vi "이벤트.vi"() -> ()   [LabVIEW 2020]
panel:
  in  "정지":bool
  in  "확인 버튼":bool
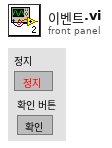
[diagram p1: front panel]
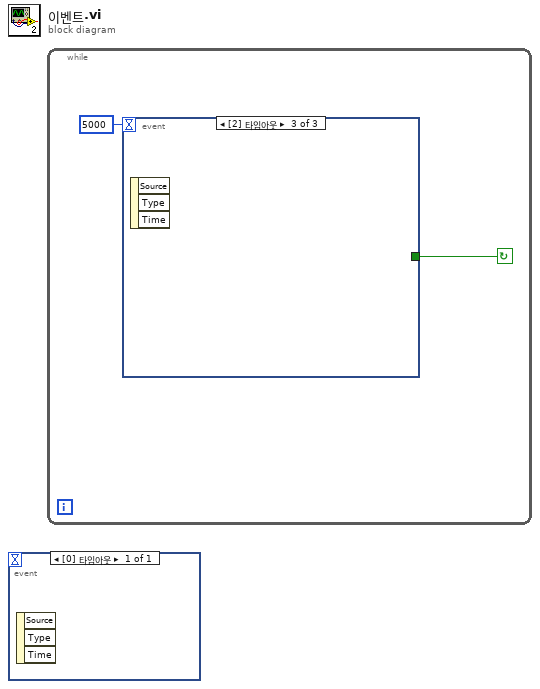
[diagram p0: block diagram]
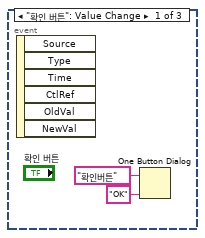
[diagram p2: hidden frame]
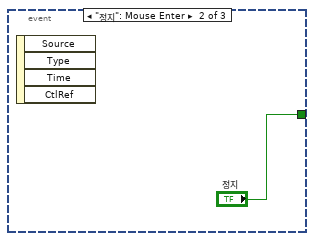
[diagram p3: hidden frame]
diagram:
  n1 = event shown="[0] 타임아웃" {
    selector: _ -> [_]
    dyn-events: _ -> [_]
    timeout: _ -> [_]
    event Timeout {
      n2 = event-data() -> ()  [unwired: 1 in, 3 out]
    }
  }
  n3 = while {
    stop <- w2 continue-if-true
    n4 = event shown="[2] 타임아웃" {
      selector: _ -> [_ _ _]
      dyn-events: _ -> [_ _ _]
      timeout: 5000 -> [_ _ _]
      tunnel: [_ "정지" _] -> w2
      event "확인 버튼": Value Change {
        n5 = event-data() -> ()  [unwired: 1 in, 6 out]
        n6 = One Button Dialog(message="확인버튼" ("메시지"), button name ("OK")="OK" ("버튼 이름(\"확인\")")) -> ()  [unwired: 1 out]
      }
      event "정지": Mouse Enter {
        n7 = event-data() -> ()  [unwired: 1 in, 4 out]
      }
      event Timeout {
        n8 = event-data() -> ()  [unwired: 1 in, 3 out]
      }
    }
  }
